vi "New Waveform Log Instance.vi"(8 "error in (no error)":errorcluster, 9 "Stop Trigger Time (optional)":timestamp, 10 "Start Trigger Time":timestamp, 11 "Waveform Log in":refnum<class "Waveform Log.lvclass">) -> (0 "error out":errorcluster, 2 "Wfm Log Instance Index":i32, 3 "Waveform Log out":refnum<class "Waveform Log.lvclass">)   [LabVIEW 2015, in "Waveform Log.lvclass"]
uses:
  Waveform Log.lvclass
  Log Instance.ctl
  Logs/Segmented Logs/Segmented Log/Segmented Log.lvclass
  Log Instance Waveform.ctl
  Waveform Information.ctl
  Waveform Data Type.ctl
  Waveform Log.lvclass/Waveform Log.ctl
  Logs/Segmented Logs/Footprint Segmented Log/Footprint Segmented Log.lvclass/Footprint Segmented Log.ctl
  Logs/Segmented Logs/Segmented Log/Segmented Log.lvclass/Segmented Log.ctl
  Logs/Segmented Logs/Segmented Log/Initialize Segmented Log.vi
  Logs/Segmented Logs/Segmented Log/Set Segmented Log Type.vi
  Logs/Segmented Logs/Footprint Segmented Log/Footprint Segmented Log.lvclass
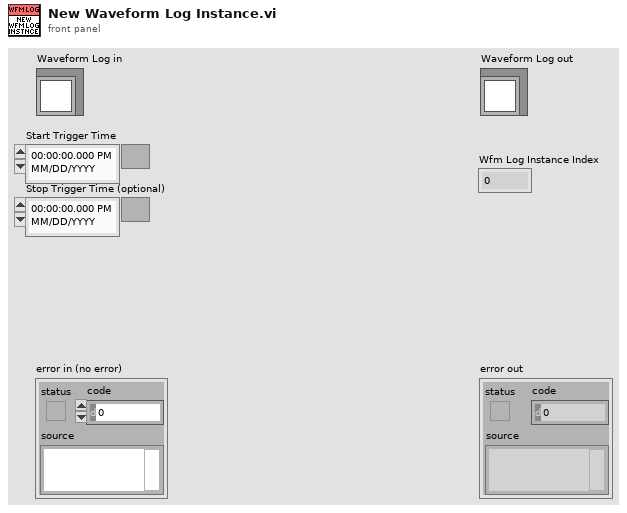
[diagram p1: front panel]
types:
  T1 = typedef "Waveform Log.lvclass/Log Instance Waveform.ctl" = cluster{"Wfm Info":T2, "Count / Instance":i32, "Previous Segment":u64, "Wfm Complete?":bool, "Last Sample Logged":timestamp, "Data Logged":bool, "Log segmented":bool}
  T2 = typedef "Waveform Log.lvclass/Waveform Information.ctl" = cluster{"Name":string, "Wfm Data Type":T3, "Decimation":u32}
  T3 = typedef "Waveform Log.lvclass/Waveform Data Type.ctl" = enum16{"Double", "ComplexDouble"}
  T4 = typedef "Waveform Log.lvclass/Log Instance.ctl" = cluster{"Segmented Log":refnum<data-value>, "Log Waveforms":T1[], "Log Start":timestamp, "Log Stop":timestamp, "Start Trigger Time":timestamp, "Stop Trigger Time":timestamp, "Time of Last Write":timestamp, "Timeout":dbl, "Stop cmd received":bool}
  T5 = typedef "Waveform Log.lvclass/Log Waveform.ctl" = cluster{"Buffer Ref":refnum<data-value>, "Wfm Info":T2}
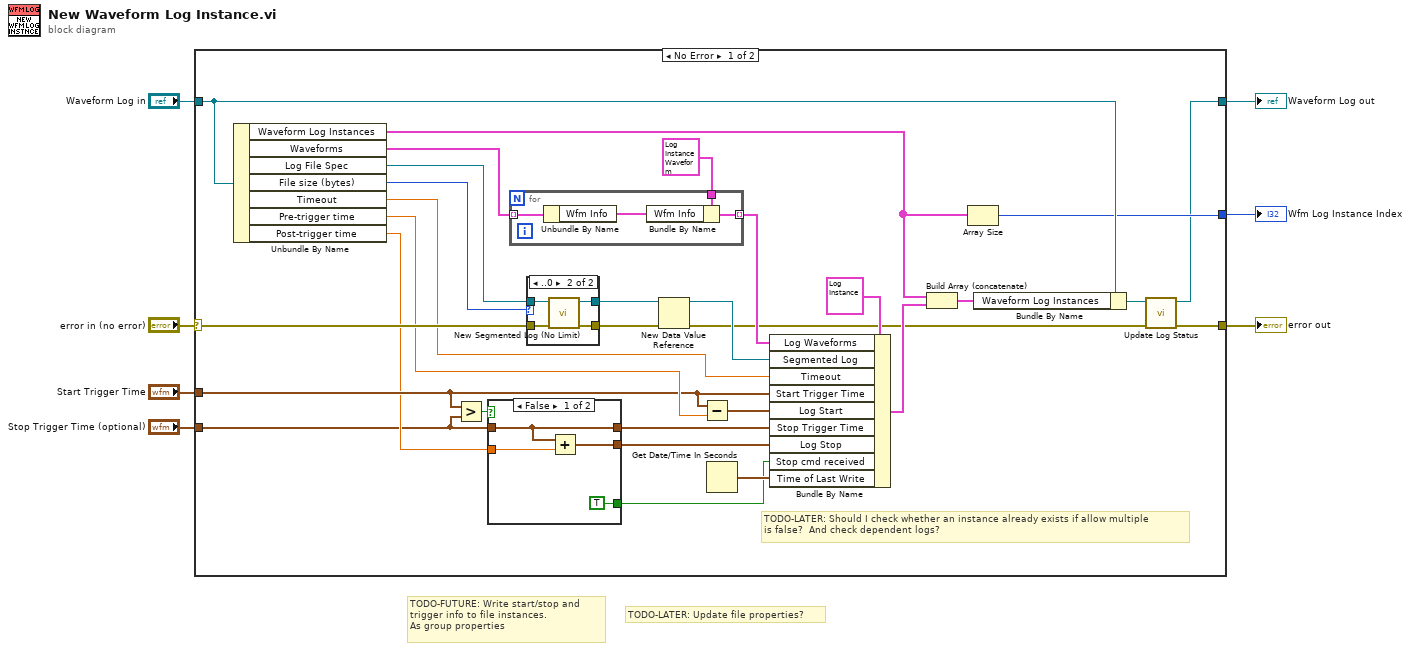
[diagram p0: block diagram]
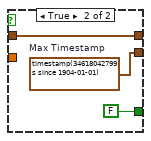
[diagram p2: hidden frame]
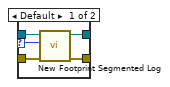
[diagram p3: hidden frame]
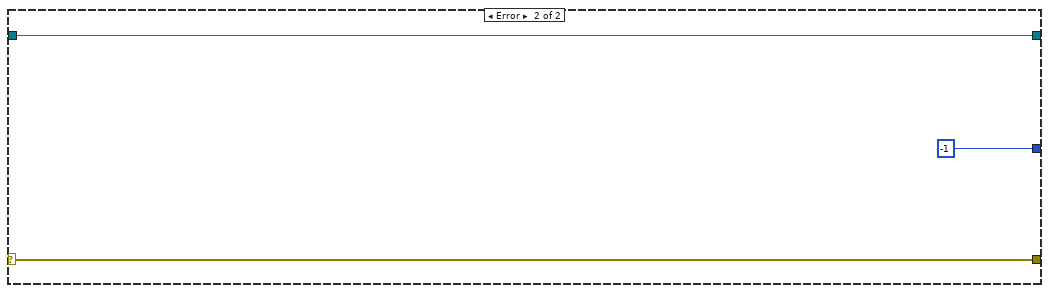
[diagram p4: hidden frame]
diagram:
  # "TODO-FUTURE: Write start/stop and \ntrigger info to file instances.\nAs group properties"
  # "TODO-LATER: Update file properties?"
  n1 = case shown="No Error" "error in (no error)" {
    selector: "error in (no error)" -> [w30 w60]
    tunnel: [w13 w60] -> w6
    tunnel: [w10 w59] -> w4
    tunnel: "Waveform Log in" -> [w36 w59]
    tunnel: "Start Trigger Time" -> [w26 _]
    tunnel: "Stop Trigger Time (optional)" -> [w22 _]
    tunnel: [w15 -1] -> w1
    frame No Error {
      # "TODO-LATER: Should I check whether an instance already exists if allow multiple\nis false?  And check dependent logs?"
      n2 = Unbundle By Name(w36) -> ("Waveform Log Instances"=w17:T4[], "Waveforms"=w35:T5[], "Log File Spec"=w19:refnum<class "Log File Specification.lvclass">, "File size (bytes)"=w18:i64, "Timeout"=w14:dbl, "Pre-trigger time"=w28:dbl, "Post-trigger time"=w24:dbl)
      n3 = Greater?(x=w26, y=w22) -> (0:w25:bool)
      n4 = case shown="False" w25 {
        tunnel: [w40 w44] -> w23
        tunnel: w22 -> [w39 w43]
        tunnel: w24 -> [w41 _]
        tunnel: [w39 w43] -> w21
        tunnel: [TRUE FALSE] -> w8
        frame False {
          n5 = Add(x=w39, y=w41) -> (x+y=w40:timestamp)
        }
        frame True {
          w44 = timestamp(34618042799 s since 1904-01-01)  # Max Timestamp
        }
      }
      n6 = for {
        tunnel: [w54] -> w33 mode=indexing
        tunnel: w35 -> [w57] mode=indexing
        tunnel: T1 {"Wfm Info"={"Name"="", "Wfm Data Type"=enum."Double", "Decimation"=0}, "Count / Instance"=0, "Previous Segment"=0, "Wfm Complete?"=FALSE, "Last Sample Logged"=timestamp(0 s since 1904-01-01), "Data Logged"=FALSE, "Log segmented"=FALSE} ("Log Waveform") -> [w56]
        n7 = Unbundle By Name(w57) -> ("Wfm Info"=w55:T2)
        n8 = Bundle By Name(cluster=w56, "Wfm Info"=w55) -> (w54:T1)
      }
      n9 = case shown="..0" w18 {
        selector: w18 -> [w46 _]
        tunnel: [w49 w53] -> w32
        tunnel: [w48 w52] -> w31
        tunnel: w30 -> [w47 w51]
        tunnel: w19 -> [w45 w50]
        frame Default {
          n10 = call "New Footprint Segmented Log.vi"("error in (no error)"=w47, "Size Limit [bytes]"=w46, "Log File Specification"=w45) -> ("error out"=w48:errorcluster, "Footprint Segmented Log out"=w49:refnum<class "Footprint Segmented Log.lvclass">)  [unwired: 7 in]
        }
        frame ..0 {
          n11 = call "New Segmented Log (No Limit).vi"("error in (no error)"=w51, "Log File Specification"=w50) -> ("error out"=w52:errorcluster, "Segmented Log out"=w53:refnum<class "Segmented Log.lvclass">)  [unwired: 8 in]
        }
      }
      n12 = New Data Value Reference(data value=w32, error in=w31) -> (data value reference=w20:refnum<data-value>, error out=w12:errorcluster)
      n13 = Subtract(x=w26, y=w28) -> (x-y=w29:timestamp)
      n14 = Get Date/Time In Seconds() -> (seconds since 1Jan1904=w9:timestamp)
      n15 = Bundle By Name(cluster=T4 {"Segmented Log"=refnum, "Log Waveforms"=[], "Log Start"=timestamp(0 s since 1904-01-01), "Log Stop"=timestamp(0 s since 1904-01-01), "Start Trigger Time"=timestamp(0 s since 1904-01-01), "Stop Trigger Time"=timestamp(0 s since 1904-01-01), "Time of Last Write"=timestamp(0 s since 1904-01-01), "Timeout"=0.0, "Stop cmd received"=FALSE} ("Log Instance"), "Log Waveforms"=w33, "Segmented Log"=w20, "Timeout"=w14, "Start Trigger Time"=w26, "Log Start"=w29, "Stop Trigger Time"=w21, "Log Stop"=w23, "Stop cmd received"=w8, "Time of Last Write"=w9) -> (w27:T4)
      n16 = Build Array (concatenate)(w17, w27) -> (w16:T4[])
      n17 = Array Size(array=w17) -> (size(s)=w15:i32)
      n18 = Bundle By Name(cluster=w36, "Waveform Log Instances"=w16) -> (w11:refnum<class "Waveform Log.lvclass">)
      n19 = call "Update Log Status.vi"("error in (no error)"=w12, "Waveform Log in"=w11) -> ("error out"=w13:errorcluster, "Waveform Log out"=w10:refnum<class "Waveform Log.lvclass">)  [unwired: 8 in]
    }
    frame Error {
    }
  }
  "error out" <- w6
  "Waveform Log out" <- w4
  "Wfm Log Instance Index" <- w1
